vi "仪器地址读取.vi"(6 "error in (no error)":errorcluster caption="错误输入（无错误）") -> (0 "error out":errorcluster caption="错误输出", 3 "仪器地址":T1)   [LabVIEW 2020]
uses:
  <vilib>/Utility/config.llb/Read Key (String).vi
  <vilib>/Utility/config.llb/NI_LVConfig.lvlib
panel:
  out "拆分的路径":path
  out "添加的路径":path
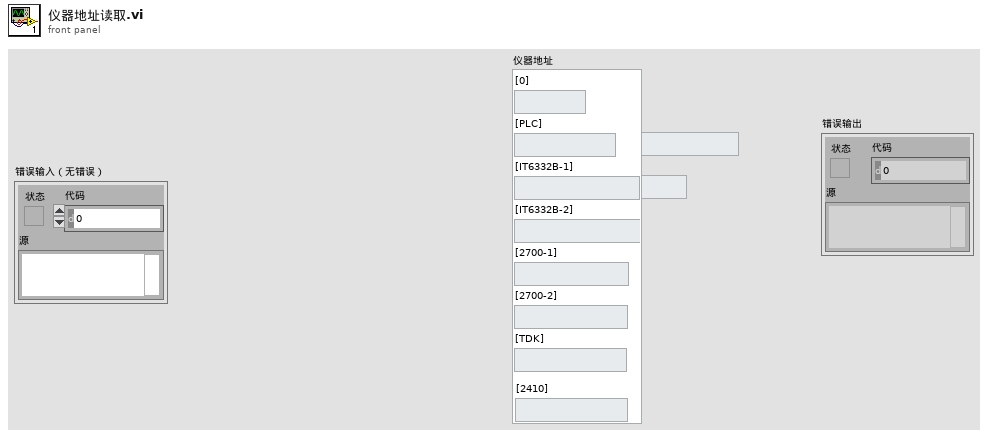
[diagram p1: front panel]
types:
  T1 = typedef "仪器地址输入.ctl" = cluster{"[0]":string, "[PLC]":string, "[IT6332B-1]":string, "[IT6332B-2]":string, "[2700-1]":string, "[2700-2]":string, "[TDK]":string, "[2410]":string}
  T2 = typedef "NI_LVConfig.lvlib/Config Data RefNum.ctl" = refnum<k1>
  T3 = cluster{"[0]":string, "[1]":string, "[2]":string, "[3]":string, "[4]":string, "[5]":string, "[6]":string, "[7]":string}
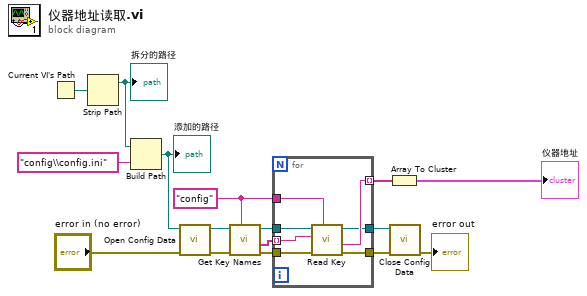
[diagram p0: block diagram]
diagram:
  w14 = "config" ("section")
  n1 = Current VI's Path() -> (path=w5:path)
  n2 = Strip Path(path=w5) -> (stripped path=w4:path)  [unwired: 1 out]
  "拆分的路径" <- w4
  n3 = Build Path(base path=w4, name or relative path="config\\config.ini") -> (appended path=w2:path)
  "添加的路径" <- w2
  n4 = call <vilib>:"Open Config Data.vi"("error in (no error)"="error in (no error)", "configuration file path"=w2) -> ("error out"=w11:errorcluster, "refnum"=w16:T2)  [unwired: 7 in, 1 out]
  n5 = call <vilib>:"Get Key Names.vi"("section"=w14, "error in (no error)"=w11, "refnum"=w16) -> ("error out"=w12:errorcluster, "key names"=w13:string[], "refnum out"=w15:T2)  [unwired: 5 in, 1 out]
  n6 = for {
    tunnel: w15 -> [w23]
    tunnel: w14 -> [w22]
    tunnel: w13 -> [w21] mode=indexing
    tunnel: w12 -> [w20]
    tunnel: [w19] -> w10 mode=indexing
    tunnel: [w18] -> w9
    tunnel: [w17] -> w8
    n7 = call-poly <vilib>:"Read Key.vi"("section"=w22, "error in (no error)"=w20, "key"=w21, "refnum"=w23) -> ("error out"=w18:errorcluster, "value"=w19:string, "refnum out"=w17:T2)  [unwired: 4 in, 1 out]
  }
  n8 = Array To Cluster(array=w10) -> (cluster=→"仪器地址":T3)
  n9 = call <vilib>:"Close Config Data.vi"("error in (no error)"=w9, "refnum"=w8) -> ("error out"=→"error out":errorcluster)  [unwired: 8 in, 1 out]
